vi "UtilityLib.guess increment from number.vi"(1 "number":dbl) -> (0 "increment":dbl)   [LabVIEW 2014, in "UtilityLib.lvlib"]
doc: "This routine guesses a proper increment value for a given number. The increment value can be used when incrementing or decrementing that number."
uses:
  UtilityLib.lvlib
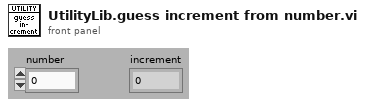
[diagram p1: front panel]
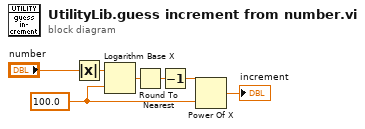
[diagram p0: block diagram]
diagram:
  w1 = 100.0 ("x")
  n1 = Absolute Value(x="number") -> (abs(x)=w5:dbl)
  n2 = Logarithm Base X(1:w1, 2:w5) -> (0:w2:dbl)
  n3 = Round To Nearest(number=w2) -> (nearest integer value=w3:dbl)
  n4 = Decrement(x=w3) -> (x-1=w4:dbl)
  n5 = Power Of X(1:w1, 2:w4) -> (0:→"increment":dbl)
